vi "Get current all controls.vi"(8 "error in (no error)":errorcluster, 11 "Sim User Console Actor in":refnum<class "Sim User Console Actor.lvclass">) -> (0 "error out":errorcluster, 3 "Sim User Console Actor out":refnum<class "Sim User Console Actor.lvclass">)   [LabVIEW 2019]
uses:
  Elevator Controller/Elevator Controller Actor Messages/Read all controls at User Console Msg/Read all controls at User Console Msg.lvclass
  <vilib>/ActorFramework/Actor/Actor.lvclass
  Floor Selection.ctl
  Sim User Console Actor.lvclass
  Door Buttons.ctl
  Elevator Call.ctl
  C:/Workspace/CLA/Elevator AF 2nd/User Console Actor/User Console Actor/User Console Actor.lvclass
  C:/Program Files (x86)/National Instruments/LabVIEW 2019/vi.lib/ActorFramework/Actor/Actor.lvclass
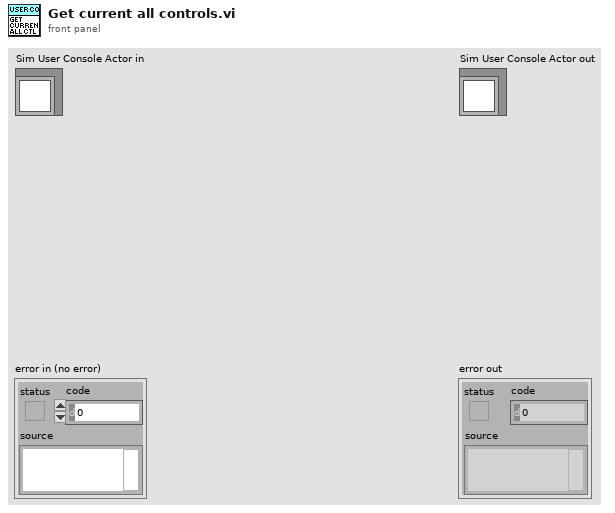
[diagram p1: front panel]
types:
  T1 = typedef "Simulated User Console Actor.lvlib/Sim User Console Actor.lvclass/Elevator Call.ctl" = cluster{"Up":bool, "Up 2":bool, "Up 3":bool, "Down":bool, "Down 2":bool, "Down 3":bool}
  T2 = typedef "Simulated User Console Actor.lvlib/Sim User Console Actor.lvclass/Door Buttons.ctl" = cluster{"Open Door":bool, "Close Door":bool}
  T3 = typedef "Simulated User Console Actor.lvlib/Sim User Console Actor.lvclass/Floor Selection.ctl" = cluster{"Floor4":bool, "Floor 3":bool, "Floor2":bool, "Floor1":bool}
  T4 = cluster{"Elevator Call":T1, "Door Buttons":T2, "Emergency":bool, "Floor Selection":T3}
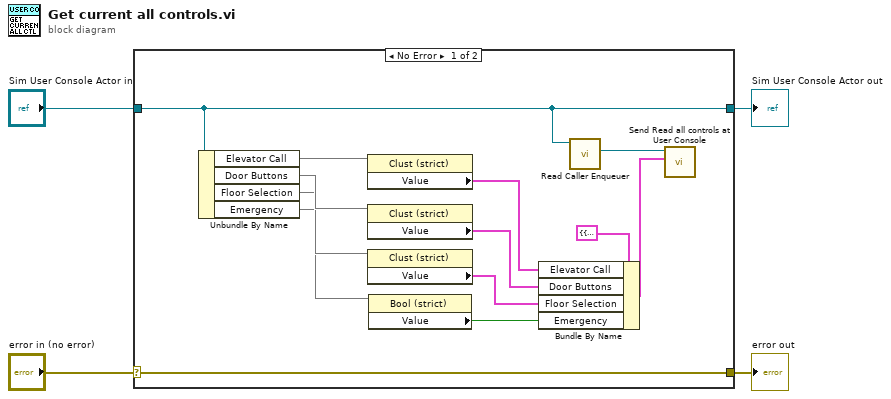
[diagram p0: block diagram]
diagram:
  n1 = case shown="No Error" "error in (no error)" {
    selector: "error in (no error)" -> [w17 w19]
    tunnel: [w17 w19] -> w3
    tunnel: [w12 w18] -> w1
    tunnel: "Sim User Console Actor in" -> [w12 w18]
    frame No Error {
      n2 = Unbundle By Name(w12) -> ("Elevator Call"=w16, "Door Buttons"=w15, "Floor Selection"=w14, "Emergency"=w13)
      n3 = property class="Clust (strict)"(reference=w16) -> ("Value"=w8:T1)  [unwired: 1 in, 2 out]
      n4 = property class="Clust (strict)"(reference=w15) -> ("Value"=w7:T2)  [unwired: 1 in, 2 out]
      n5 = property class="Clust (strict)"(reference=w14) -> ("Value"=w6:T3)  [unwired: 1 in, 2 out]
      n6 = property class="Bool (strict)"(reference=w13) -> ("Value"=w5:bool)  [unwired: 1 in, 2 out]
      n7 = Bundle By Name(cluster=T4 {"Elevator Call"={"Up"=FALSE, "Up 2"=FALSE, "Up 3"=FALSE, "Down"=FALSE, "Down 2"=FALSE, "Down 3"=FALSE}, "Door Buttons"={"Open Door"=FALSE, "Close Door"=FALSE}, "Emergency"=FALSE, "Floor Selection"={"Floor4"=FALSE, "Floor 3"=FALSE, "Floor2"=FALSE, "Floor1"=FALSE}} ("All controls"), "Elevator Call"=w8, "Door Buttons"=w7, "Floor Selection"=w6, "Emergency"=w5) -> (w9:T4)
      n8 = call <vilib>:"Read Caller Enqueuer.vi"("Actor"=w12) -> ("Caller Enqueuer"=w11:refnum<class "Message Enqueuer.lvclass">)  [unwired: 10 in]
      n9 = call "Send Read all controls at User Console.vi"("All controls"=w9, "Message Enqueuer"=w11) -> ()  [unwired: 8 in, 2 out]
    }
    frame Error {
    }
  }
  "error out" <- w3
  "Sim User Console Actor out" <- w1
